vi "GA_Insert Into Population.vi"(6 "Parameters":T3={"Population size"=100, "Generations no."=500, "Crossover probabality"=6.0, "Mutation mode"=enum."one-point, fitness-adjustable rate", "Creep mutation"=FALSE, "Mutation rate"=0.005, "Min mutation rate"=0.005, "Max mutation rate"=0.0005, "Relative fitness differential"=0.25, "Reproduction plan"=enum."Steady-state-replace-random", "Elitism"=FALSE, "FeaturesPerChannel"=0} {"Relative fitness differential" min=0.0 max=1.0; "Max mutation rate" min=0.0 max=1.0; "Min mutation rate" min=0.0 max=1.0; "Mutation rate" min=0.0 max=1.0; "Crossover probabality" min=0.0 max=1.0; "Generations no." min=1; "Population size" min=1}, 7 "Fitness Function":T2, 9 "Offsprings":i8[][](array[numeric]), 11 "Population in":T1) -> (3 "Population out":T1)   [LabVIEW 2016, in "GA.lvlib"]
doc: "Inserts children in proper place into population taking care about reproduction plan and elitism.\nOnly for steady-state reproduction plans"
uses:
  GA.lvlib
  GA_tParameters.ctl
  GA_tFitness Function.ctl
  4. Accuracy Assessment for EEG Classification/_vlib/ClassifierClass.lvclass
  GA_tPopulation.ctl
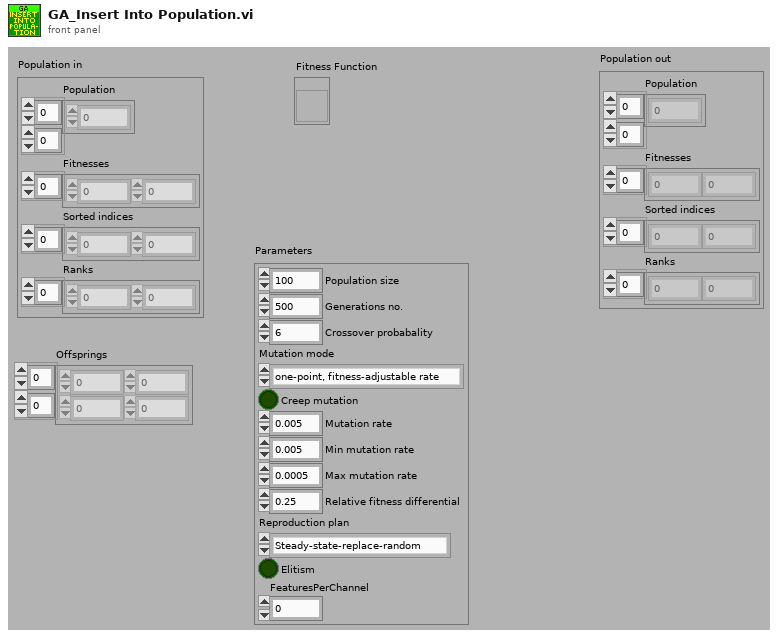
[diagram p1: front panel]
types:
  T1 = typedef "GA.lvlib/GA_tPopulation.ctl" = cluster{"Population":i8[][], "Fitnesses":dbl[], "Sorted indices":i32[], "Ranks":i32[]}
  T2 = typedef "GA.lvlib/GA_tFitness Function.ctl" = refnum<vi>
  T3 = typedef "GA.lvlib/GA_tParameters.ctl" = cluster{"Population size":i32, "Generations no.":i32, "Crossover probabality":dbl, "Mutation mode":enum16{"one-point, fixed rate", "one-point, fitness-adjustable rate", "one-point, distance-adjustable rate"}, "Creep mutation":bool, "Mutation rate":dbl, "Min mutation rate":dbl, "Max mutation rate":dbl, "Relative fitness differential":dbl, "Reproduction plan":enum16{"Full generational replacement", "Steady-state-replace-random", "Steady-state-replace-worst"}, "Elitism":bool, "FeaturesPerChannel":i32}
  T4 = enum16{"Full generational replacement", "Steady-state-replace-random", "Steady-state-replace-worst"}
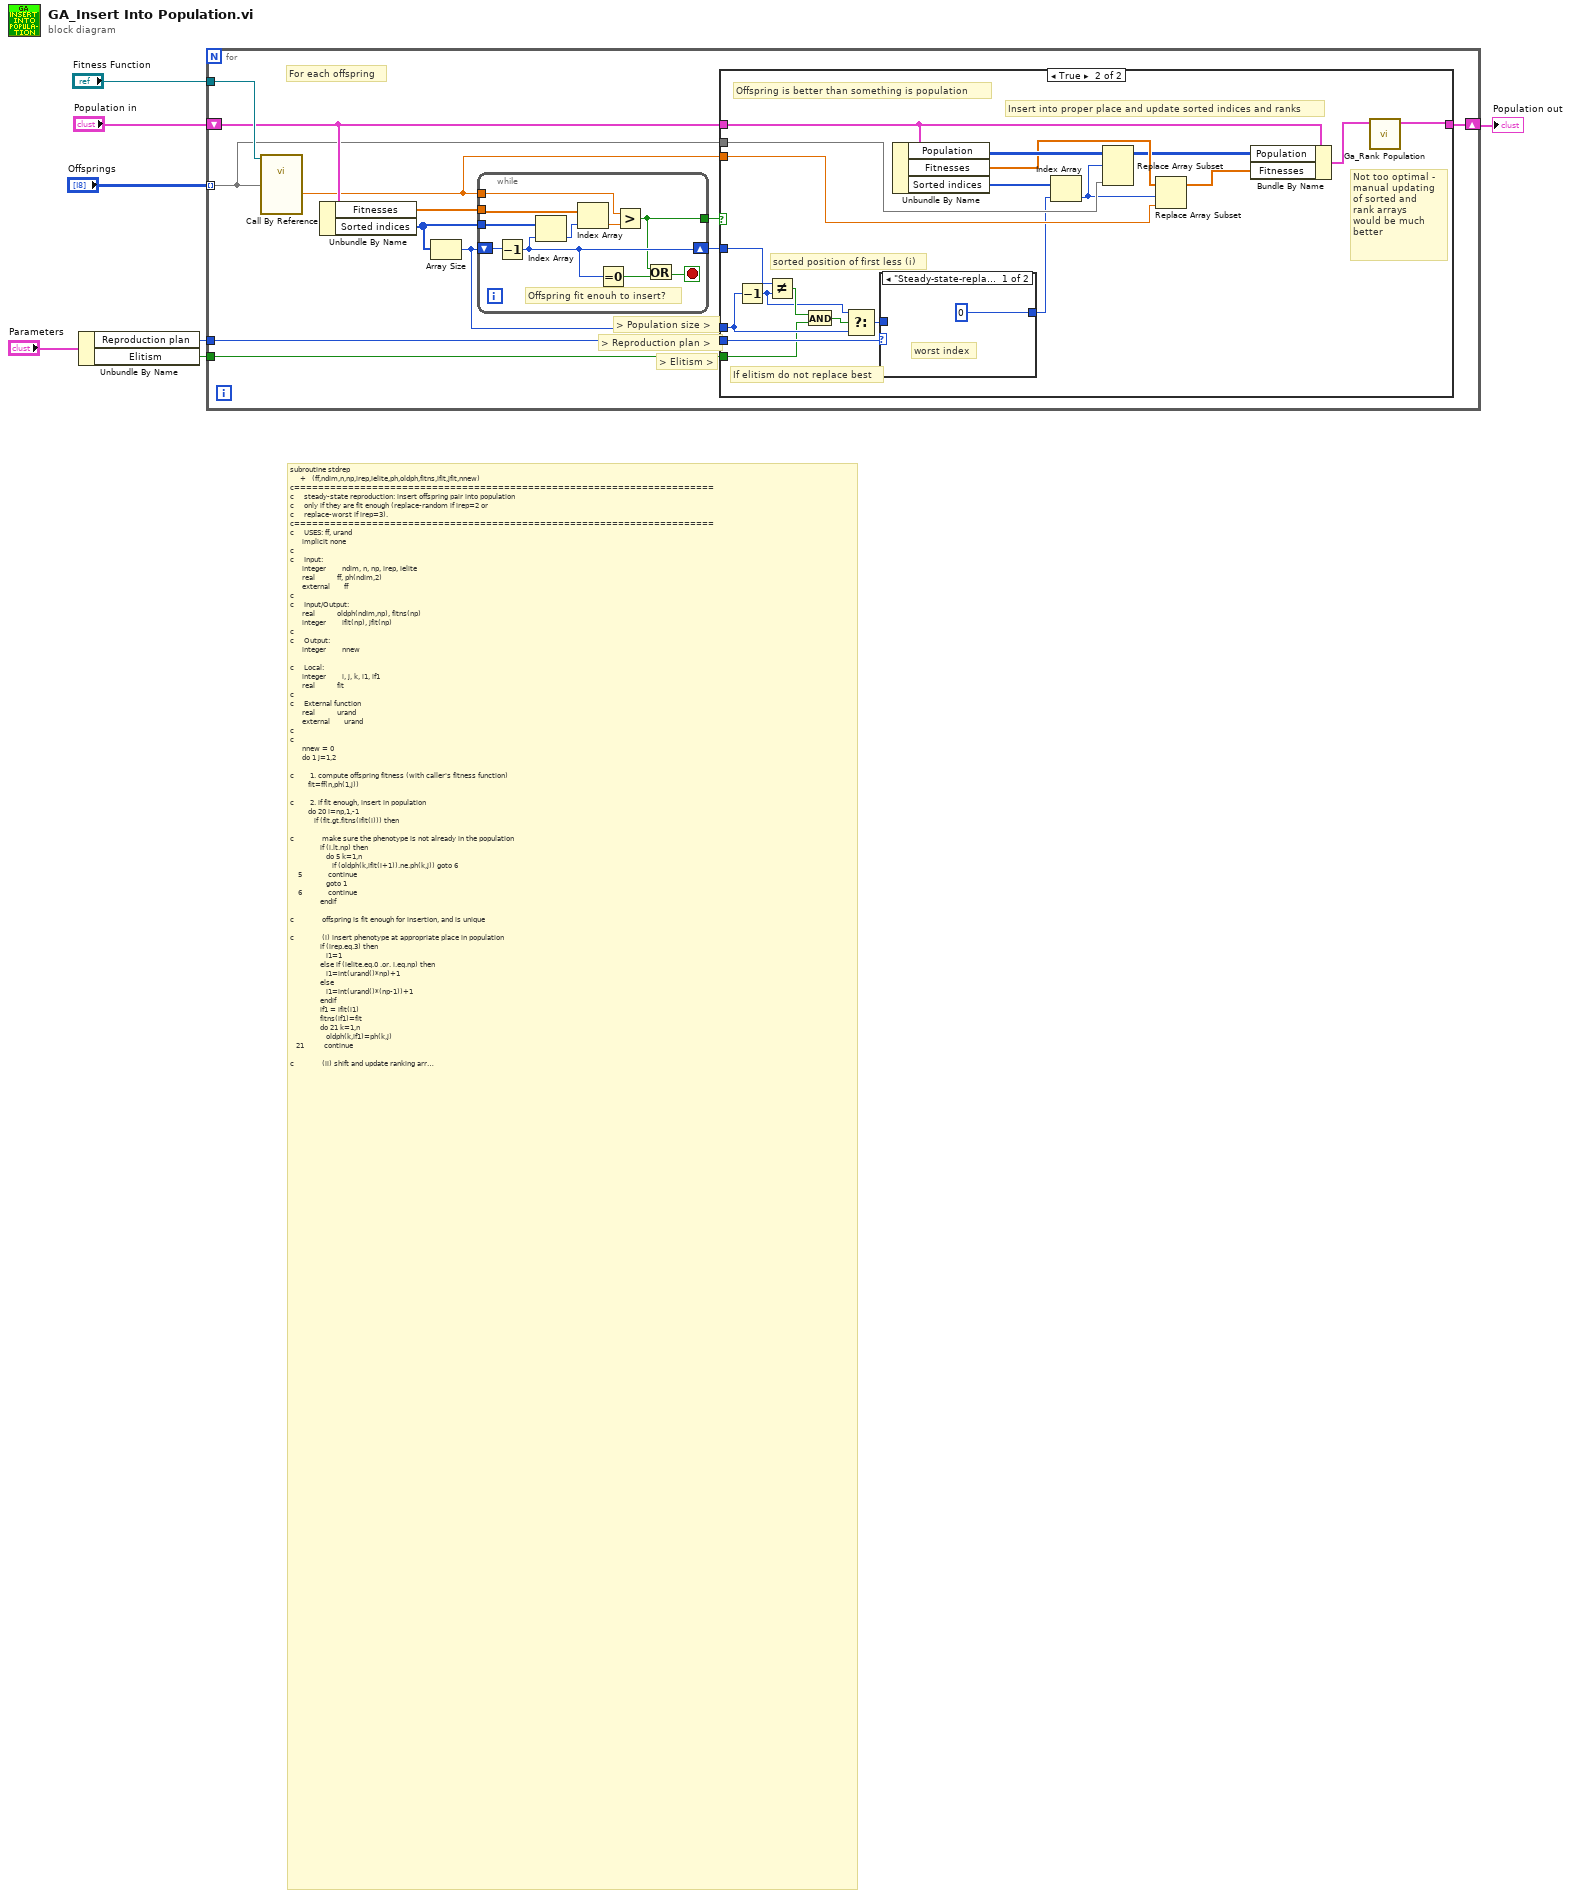
[diagram p0: block diagram]
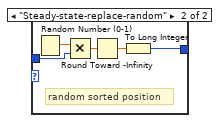
[diagram p3: hidden frame]
diagram:
  # "subroutine stdrep\n     +   (ff,ndim,n,np,irep,ielite,ph,oldph,fitns,ifit,jfit,nnew)\nc======================================================================\nc     steady-state reproduction: insert offspring pair into population\nc     only if they are fit enough (replace-random if irep=2 or\nc     replace-worst if irep=3).\nc======================================================================\nc     USES: ff, urand\n      implicit none\nc\nc     Input:\n      integer        ndim, n, np, irep, ielite\n      real           ff, ph(ndim,2)\n      external       ff\nc\nc     Input/Output:\n      real           oldph(ndim,np), fitns(np)\n      integer        ifit(np), jfit(np)\nc\nc     Output:\n      integer        nnew\n \nc     Local:\n      integer        i, j, k, i1, if1\n      real           fit\nc\nc     External function\n      real           urand\n      external       urand\nc\nc\n      nnew = 0\n      do 1 j=1,2\n \nc        1. compute offspring fitness (with caller's fitness function)\n         fit=ff(n,ph(1,j))\n \nc        2. if fit enough, insert in population\n         do 20 i=np,1,-1\n            if (fit.gt.fitns(ifit(i))) then\n \nc              make sure the phenotype is not already in the population\n               if (i.lt.np) then\n                  do 5 k=1,n\n                     if (oldph(k,ifit(i+1)).ne.ph(k,j)) goto 6\n    5             continue\n                  goto 1\n    6             continue\n               endif\n \nc              offspring is fit enough for insertion, and is unique\n \nc              (i) insert phenotype at appropriate place in population\n               if (irep.eq.3) then\n                  i1=1\n               else if (ielite.eq.0 .or. i.eq.np) then\n                  i1=int(urand()*np)+1\n               else\n                  i1=int(urand()*(np-1))+1\n               endif\n               if1 = ifit(i1)\n               fitns(if1)=fit\n               do 21 k=1,n\n                  oldph(k,if1)=ph(k,j)\n   21          continue\n \nc              (ii) shift and update ranking arrays\n               if (i.lt.i1) then\n \nc                 shift up\n                  jfit(if1)=np-i\n                  do 22 k=i1-1,i+1,-1\n                     jfit(ifit(k))=jfit(ifit(k))-1\n                     ifit(k+1)=ifit(k)\n   22             continue\n                  ifit(i+1)=if1\n               else\n \nc                 shift down\n                  jfit(if1)=np-i+1\n                  do 23 k=i1+1,i\n                     jfit(ifit(k))=jfit(ifit(k))+1\n                     ifit(k-1)=ifit(k)\n   23             continue\n                  ifit(i)=if1\n               endif\n               nnew = nnew+1\n               goto 1\n            endif\n   20    continue\n \n    1 continue\n \n      return\n      end"
  n1 = Unbundle By Name("Parameters") -> ("Reproduction plan"=w4:T4, "Elitism"=w2:bool)
  n2 = for {
    tunnel: "Offsprings" -> [w13] mode=indexing
    shift-right: [w8] -> w1
    shift-left: "Population in" -> [w15]
    tunnel: w4 -> [w12]
    tunnel: "Fitness Function" -> [w19]
    tunnel: w2 -> [w10]
    # "> Population size >"
    # "> Elitism >"
    # "> Reproduction plan >"
    # "For each offspring"
    n3 = call-by-ref "?"(reference=w19, "Phenotype"=w13) -> ("Fitness"=w14:dbl)  [unwired: 3 in, 2 out]
    n4 = Unbundle By Name(w15) -> ("Fitnesses"=w18:dbl[], "Sorted indices"=w17:i32[])
    n5 = Array Size(array=w17) -> (size(s)=w11:i32)
    n6 = while {
      tunnel: w18 -> [w54]
      tunnel: w17 -> [w55]
      shift-right: [w53] -> w9
      shift-left: w11 -> [w56]
      tunnel: w14 -> [w51]
      tunnel: [w48] -> w16
      stop <- w49 stop-if-true
      # "Offspring fit enouh to insert?"
      n7 = Decrement(x=w56) -> (x-1=w53:i32)
      n8 = Index Array(array=w55, index=w53) -> (element=w47:i32)
      n9 = Index Array(array=w54, index=w47) -> (element=w52:dbl)
      n10 = Equal To 0?(x=w53) -> (x = 0?=w50:bool)
      n11 = Greater?(x=w51, y=w52) -> (0:w48:bool)
      n12 = Or(x=w48, y=w50) -> (x .or. y?=w49:bool)
    }
    n13 = case shown="True" w16 {
      tunnel: w15 -> [w20 w30]
      tunnel: w14 -> [_ w36]
      tunnel: w13 -> [_ w38]
      tunnel: w12 -> [_ w40]
      tunnel: w11 -> [_ w32]
      tunnel: w9 -> [_ w26]
      tunnel: w10 -> [_ w23]
      tunnel: [w20 w24] -> w8
      frame False {
        # "Offspring is worse than whole population"
      }
      frame True {
        # "Offspring is better than something is population"
        # "Not too optimal -\nmanual updating\nof sorted and\nrank arrays\nwould be much\nbetter"
        # "If elitism do not replace best"
        # "Insert into proper place and update sorted indices and ranks"
        # "sorted position of first less (i)"
        n14 = Decrement(x=w32) -> (x-1=w21:i32)
        n15 = Not Equal?(x=w26, y=w21) -> (x != y?=w34:bool)
        n16 = And(x=w34, y=w23) -> (x .and. y?=w33:bool)
        n17 = Select(t=w21, s=w33, f=w32) -> (s? t:f=w31:i32)
        n18 = case shown="\"Steady-state-replace-worst\", Default" w40 {
          tunnel: w31 -> [_ w45]
          tunnel: [0 w42] -> w22
          frame "Steady-state-replace-worst", Default {
            # "worst index"
          }
          frame "Steady-state-replace-random" {
            # "random sorted position"
            n19 = Random Number (0-1)() -> (number: 0 to 1=w46:dbl)
            n20 = Multiply(x=w46, y=w45) -> (x*y=w44:dbl)
            n21 = Round Toward -Infinity(1:w44) -> (0:w43:dbl)
            n22 = To Long Integer(number=w43) -> (32bit integer=w42:i32)
          }
        }
        n23 = Unbundle By Name(w30) -> ("Population"=w39:i8[][], "Fitnesses"=w37:dbl[], "Sorted indices"=w35:i32[])
        n24 = Index Array(array=w35, index=w22) -> (element=w27:i32)
        n25 = Replace Array Subset(array=w39, new element=w38, index (row)=w27) -> (w29:i8[][])  [unwired: 1 in]
        n26 = Replace Array Subset(array=w37, new element=w36, index=w27) -> (w28:dbl[])
        n27 = Bundle By Name(cluster=w30, "Population"=w29, "Fitnesses"=w28) -> (w25:T1)
        n28 = call "Ga_Rank Population.vi"("Population in"=w25) -> ("Population out"=w24:T1)  [unwired: 10 in]
      }
    }
  }
  "Population out" <- w1
